vi "ValveStub.vi"(8 "error in":errorcluster, 10 "ON":bool=TRUE, 11 "Valve":u16=999) -> (0 "error out":errorcluster)   [LabVIEW 2012]
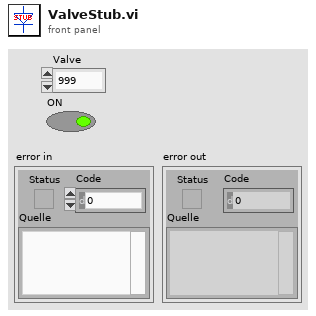
[diagram p1: front panel]
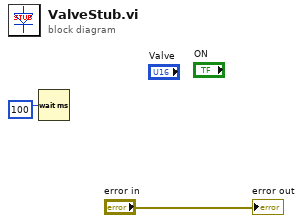
[diagram p0: block diagram]
diagram:
  n1 = Wait (ms)(milliseconds to wait=100) -> ()  [unwired: 1 out]
  "error out" <- "error in"
